vi "PwF_ToF_DeviceID_Tuning_Panel.vi"() -> ()   [LabVIEW 2018]
panel:
  in  "Flash LED of Device per SN below":bool
  out "Device ID Matches Desired":bool
  in  "Device Reconfigure Command":bool
  in  "Desired Device ID":u8
  in  "Serial No of Device to Config":u32
  out "ToF Device List":u32[][](array[numeric])
  # "Playing With Fusion Time of Flight Sensor"
  # "Purpose:\nUse this VI to \n     a) detect Playing With Fusion ToF devices connected to the datalink\n     b) Configure the device ID for the device of your choice, based on the unique Hardware Serial Number of said device \nDrop this VI in a while loop with a quick (50ms or faster recommended) update rate and run. The ToF device list will populate\nas additioanl devices are seen communicating on the link. You will use the Device List table to identify your device and to \nverify that your device has been successfully configured. It may take 10-30 seconds for all connected devices to show up\nin the table., so please be patient."
  # "List of ToF Devices Detected on Bus\nNote: Ignore entry with all zeroes"
  # "HW Serial Number"
  # "Device ID (should be different)"
  # "Manuf ID"
  # "Firmware Rev"
  # "To change device ID:\n1) Look above to identify the Serial Number (first row of table) of the device you want to change\n2) Enter that serial number in the box below\n3) Press \"Flash LED\" button to make sure you're configuring the correct device (device LED will blink)\n4) Enter the new Device ID you'd like to select (0-255)\n5) Press the Button once to trigger a reconfiguration request\n6) Check the device list above to verify that the Device ID of the ToF device you selected has changed\n     - note: this may take a few seconds to show up"
  # "<---- This will light up if the desired ID of the specified \ndevice matches what the device is broadcasting on"
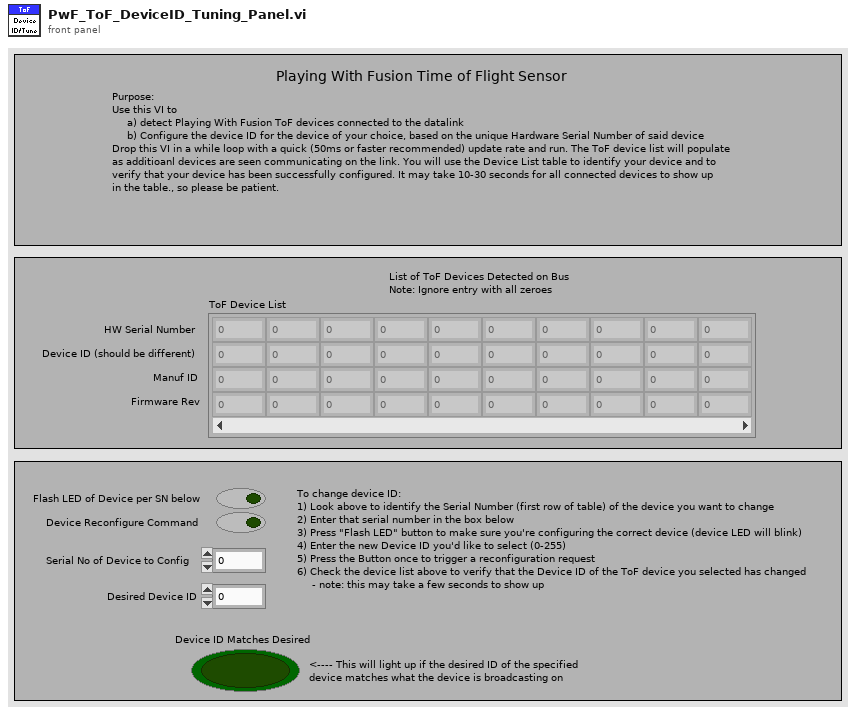
[diagram p1: front panel]
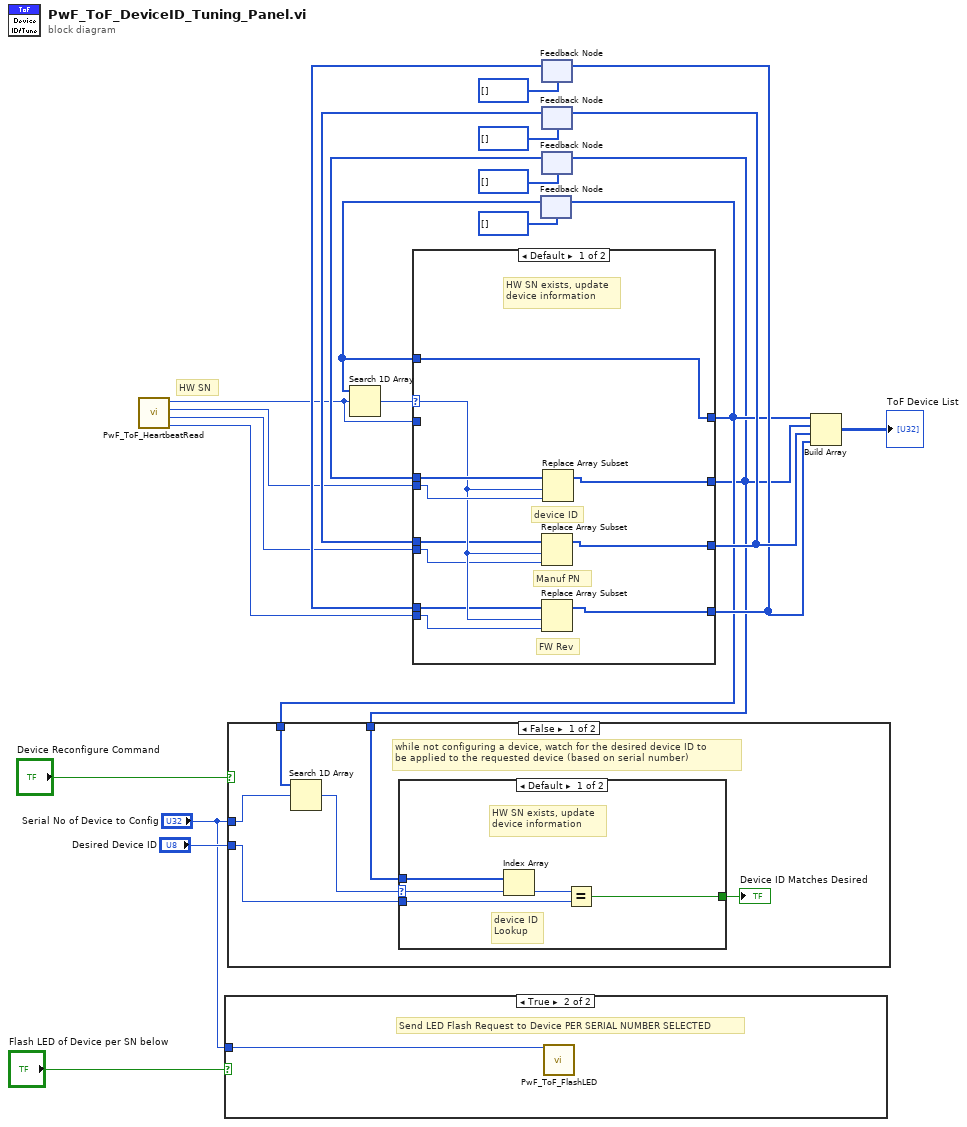
[diagram p0: block diagram]
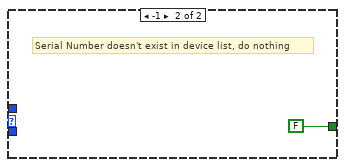
[diagram p3: hidden frame]
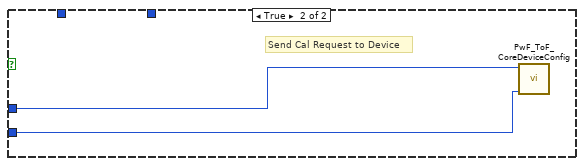
[diagram p4: hidden frame]
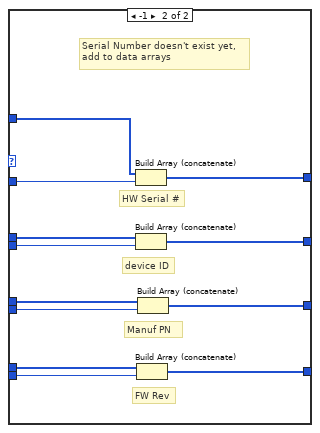
[diagram p5: hidden frame]
diagram:
  # "HW SN"
  n1 = call "PwF_ToF_HeartbeatRead.vi"() -> ("Firmware Rev"=w7:u16, "Manuf PN"=w8:u16, "Device ID"=w9:u8, "Hardware SN"=w10:u32)  [unwired: 8 in]
  n2 = case shown="True" "Flash LED of Device per SN below" {
    tunnel: "Serial No of Device to Config" -> [_ w23]
    frame False {
    }
    frame True {
      # "Send LED Flash Request to Device PER SERIAL NUMBER SELECTED"
      n3 = call "PwF_ToF_FlashLED.vi"("HW Serial Number"=w23) -> ()  [unwired: 14 in, 1 out]
    }
  }
  n4 = feedback #1(u32[] []) -> (w21:u32[])
  n5 = Search 1D Array(1D array=w21, element=w10) -> (index of element=w22:i32)  [unwired: 1 out]
  n6 = feedback #2(u16[] []) -> (w17:u16[])
  n7 = feedback #3(u16[] []) -> (w18:u16[])
  n8 = feedback #4(u8[] []) -> (w20:u8[])
  n9 = case shown="Default" w22 {
    selector: w22 -> [w30 _]
    tunnel: [w34 w46] -> w5
    tunnel: w21 -> [w34 w45]
    tunnel: w10 -> [_ w44]
    tunnel: [w31 w43] -> w3
    tunnel: w20 -> [w33 w42]
    tunnel: w9 -> [w32 w41]
    tunnel: w8 -> [w24 w40]
    tunnel: [w25 w39] -> w14
    tunnel: w18 -> [w26 w38]
    tunnel: w7 -> [w29 w37]
    tunnel: [w28 w36] -> w13
    tunnel: w17 -> [w27 w35]
    frame Default {
      # "FW Rev"
      # "Manuf PN"
      # "device ID"
      # "HW SN exists, update\ndevice information"
      n10 = Replace Array Subset(array=w26, new element=w24, index=w30) -> (w25:u16[])
      n11 = Replace Array Subset(array=w27, new element=w29, index=w30) -> (w28:u16[])
      n12 = Replace Array Subset(array=w33, new element=w32, index=w30) -> (w31:u8[])
    }
    frame -1 {
      # "FW Rev"
      # "Manuf PN"
      # "HW Serial #"
      # "device ID"
      # "Serial Number doesn't exist yet,\nadd to data arrays"
      n13 = Build Array (concatenate)(w45, w44) -> (w46:u32[])
      n14 = Build Array (concatenate)(w42, w41) -> (w43:u8[])
      n15 = Build Array (concatenate)(w35, w37) -> (w36:u16[])
      n16 = Build Array (concatenate)(w38, w40) -> (w39:u16[])
    }
  }
  n17 = case shown="False" "Device Reconfigure Command" {
    tunnel: w5 -> [w52 _]
    tunnel: "Desired Device ID" -> [w47 w60]
    tunnel: "Serial No of Device to Config" -> [w51 w59]
    tunnel: w3 -> [w48 _]
    frame False {
      # "while not configuring a device, watch for the desired device ID to \nbe applied to the requested device (based on serial number)"
      n18 = Search 1D Array(1D array=w52, element=w51) -> (index of element=w49:i32)  [unwired: 1 out]
      n19 = case shown="Default" w49 {
        selector: w49 -> [w53 _]
        tunnel: [w56 FALSE] -> w50
        tunnel: w48 -> [w55 _]
        tunnel: w47 -> [w57 _]
        frame Default {
          # "device ID\nLookup"
          # "HW SN exists, update\ndevice information"
          n20 = Index Array(array=w55, index=w53) -> (element=w54:u8)
          n21 = Equal?(x=w54, y=w57) -> (x = y?=w56:bool)
        }
        frame -1 {
          # "Serial Number doesn't exist in device list, do nothing"
        }
      }
      "Device ID Matches Desired" <- w50
    }
    frame True {
      # "Send Cal Request to Device"
      n22 = call "PwF_ToF_CoreDeviceConfig.vi"("NewDeviceID"=w60, "SNofDevToChange"=w59) -> ()  [unwired: 10 in]
    }
  }
  n23 = feedback-in #1(w5) -> ()
  n24 = feedback-in #2(w13) -> ()
  n25 = feedback-in #3(w14) -> ()
  n26 = feedback-in #4(w3) -> ()
  n27 = Build Array(w5, w3, w14, w13) -> (→"ToF Device List":u32[][])
